vi "LaneExtractorHenes.vi"() -> ()   [LabVIEW 2024]
uses:
  <vilib>/userDefined/High Color/IMAQdx.ctl
  <vilib>/Instr/_visa.llb/VISA Set IO Buffer Mask.ctl
  <vilib>/Instr/_visa.llb/VISA Flush IO Buffer Mask.ctl
  <vilib>/Python/Open Venv Python Session.vi
  <vilib>/Instr/_visa.llb/VISA Configure Serial Port (Instr).vi
  <vilib>/vision/driver/NI_Vision_Acquisition_Software.lvlib
panel:
  out "inference time":string
  out "error out 3":errorcluster
  out "Image_String":string
  in  "File Path":path=path "C:/Users/JungiHong/OneDrive/Hongik/HI-RACE/2026-01/platform_1_5/ExperimentModules/LaneTracking/forTrainImages/frame_021.jpg"
  in  "UseVideo":bool
  in  "Cam No.":T1="cam3"
  out "Debug":T2(plugin-control)
  in  "input_spd":i16
  in  "HENES":refnum<visa-resource-name>="COM5"
  out "E-STOP":bool
  out "Remote_M/A":bool
  out "Steer_Feed":dbl
  out "Alive_PCU":u8(slide) scale=0.0..254.0
  out "Gear_Feed":u8
  out "Speed_Feed(RPM)":dbl format="%#_g rpm"
  out "버퍼 읽기":string
  out "Speed_Feed(m/s)":dbl
  in  "HLV_Gear":u8
  in  "HLV_A/M":bool=TRUE
  in  "HLV_E-stop":bool
  out "HENES Loop Time":u32=21
  in  "v(Velocity)m/s":dbl=1.0
  in  "k(Gain)":dbl=1.0
  out "δ(OutputSteer)degrees":dbl=6.391264837490994
  in  "max_rmse":u32=1000
  in  "min_span":u32=4
  in  "min_area":u32=4
  out "Right":T2(plugin-control)
  out "changearray":u32=3
  out "CV Loop Time":u32=32
  out "error out 2":errorcluster
  out "error out":errorcluster
  out "return value":string[](array[string])=["0.0", "0.11201359920254694", "C:\\Users\\JungiHong\\OneDrive\\Hongik\\HI-RACE\\2026-01\\platform_1_5\\ExperimentModules\\LaneTracking\\DebugImageFolder\\left_lane.png", "C:\\Users\\JungiHong\\OneDrive\\Hongik\\HI-RACE\\2026-01\\platform_1_5\\ExperimentModules\\LaneTracking\\DebugImageFolder\\right_lane.png", "C:\\Users\\JungiHong\\OneDrive\\Hongik\\HI-RACE\\2026-01\\platform_1_5\\ExperimentModules\\LaneTracking\\DebugImageFolder\\debug_image.png"]
  out "python_error":errorcluster
  out "Left":T2(plugin-control)
  in  "stop":bool
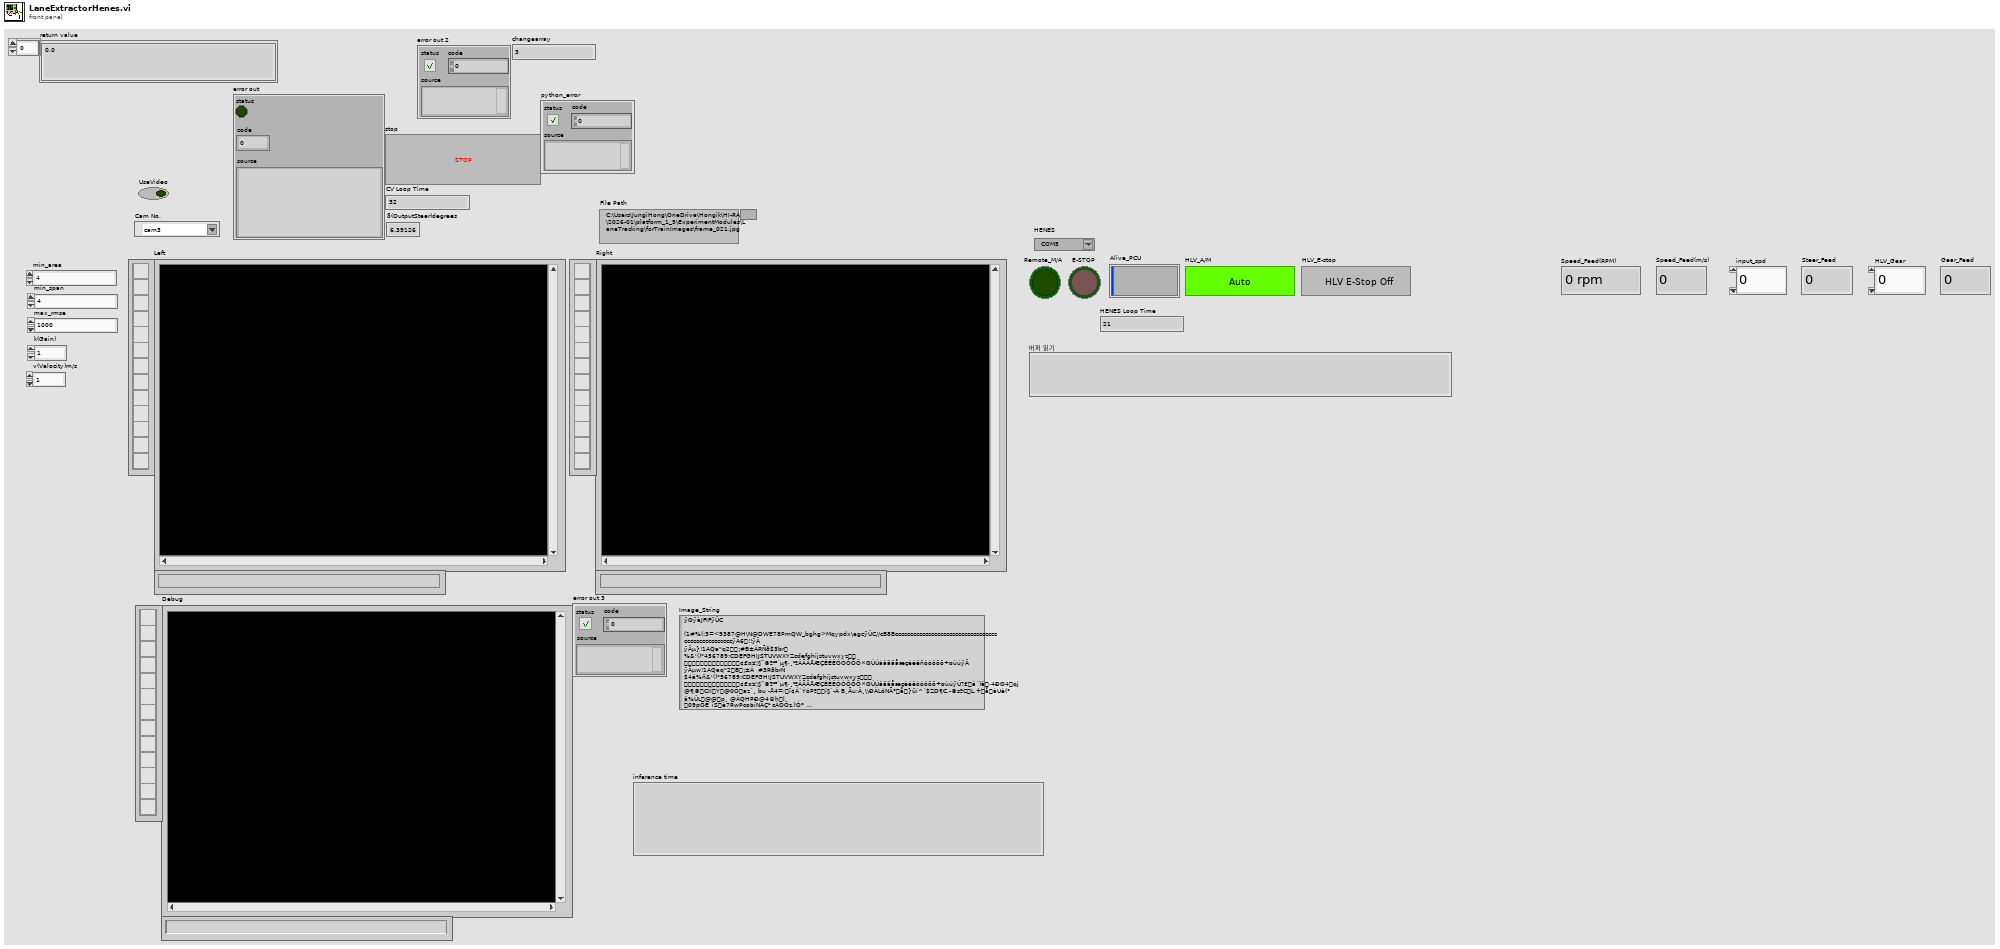
[diagram p1: front panel]
types:
  T1 = typedef "IMAQdx.ctl" = refnum<k21>
  T2 = typedef "IMAQ Image.ctl" = refnum<image>
  T3 = cluster{"HENES_M/A":u8, "HENES_E-Stop":u8, "HENES_Gear":u8, "HENES_Speed":i16, "HENES_Steer":i16, "HENES_Alive":u8}
  T4 = typedef "VISA Flush IO Buffer Mask.ctl" = u16
  T5 = typedef "VISA Set IO Buffer Mask.ctl" = u16
  T6 = cluster{"HLV_M/A_Status":u8, "HLV_E-Stop":u8, "HLV_Gear":u8, "HLV_Speed":i16, "HLV_Steer":i16, "HLV_Alive":u8}
  T7 = cluster{"Global Rectangle":i32[], "Contours":cluster{"ID":enum32{"External", "Internal"}, "Type":u32, "Coordinates":i32[]}[]}
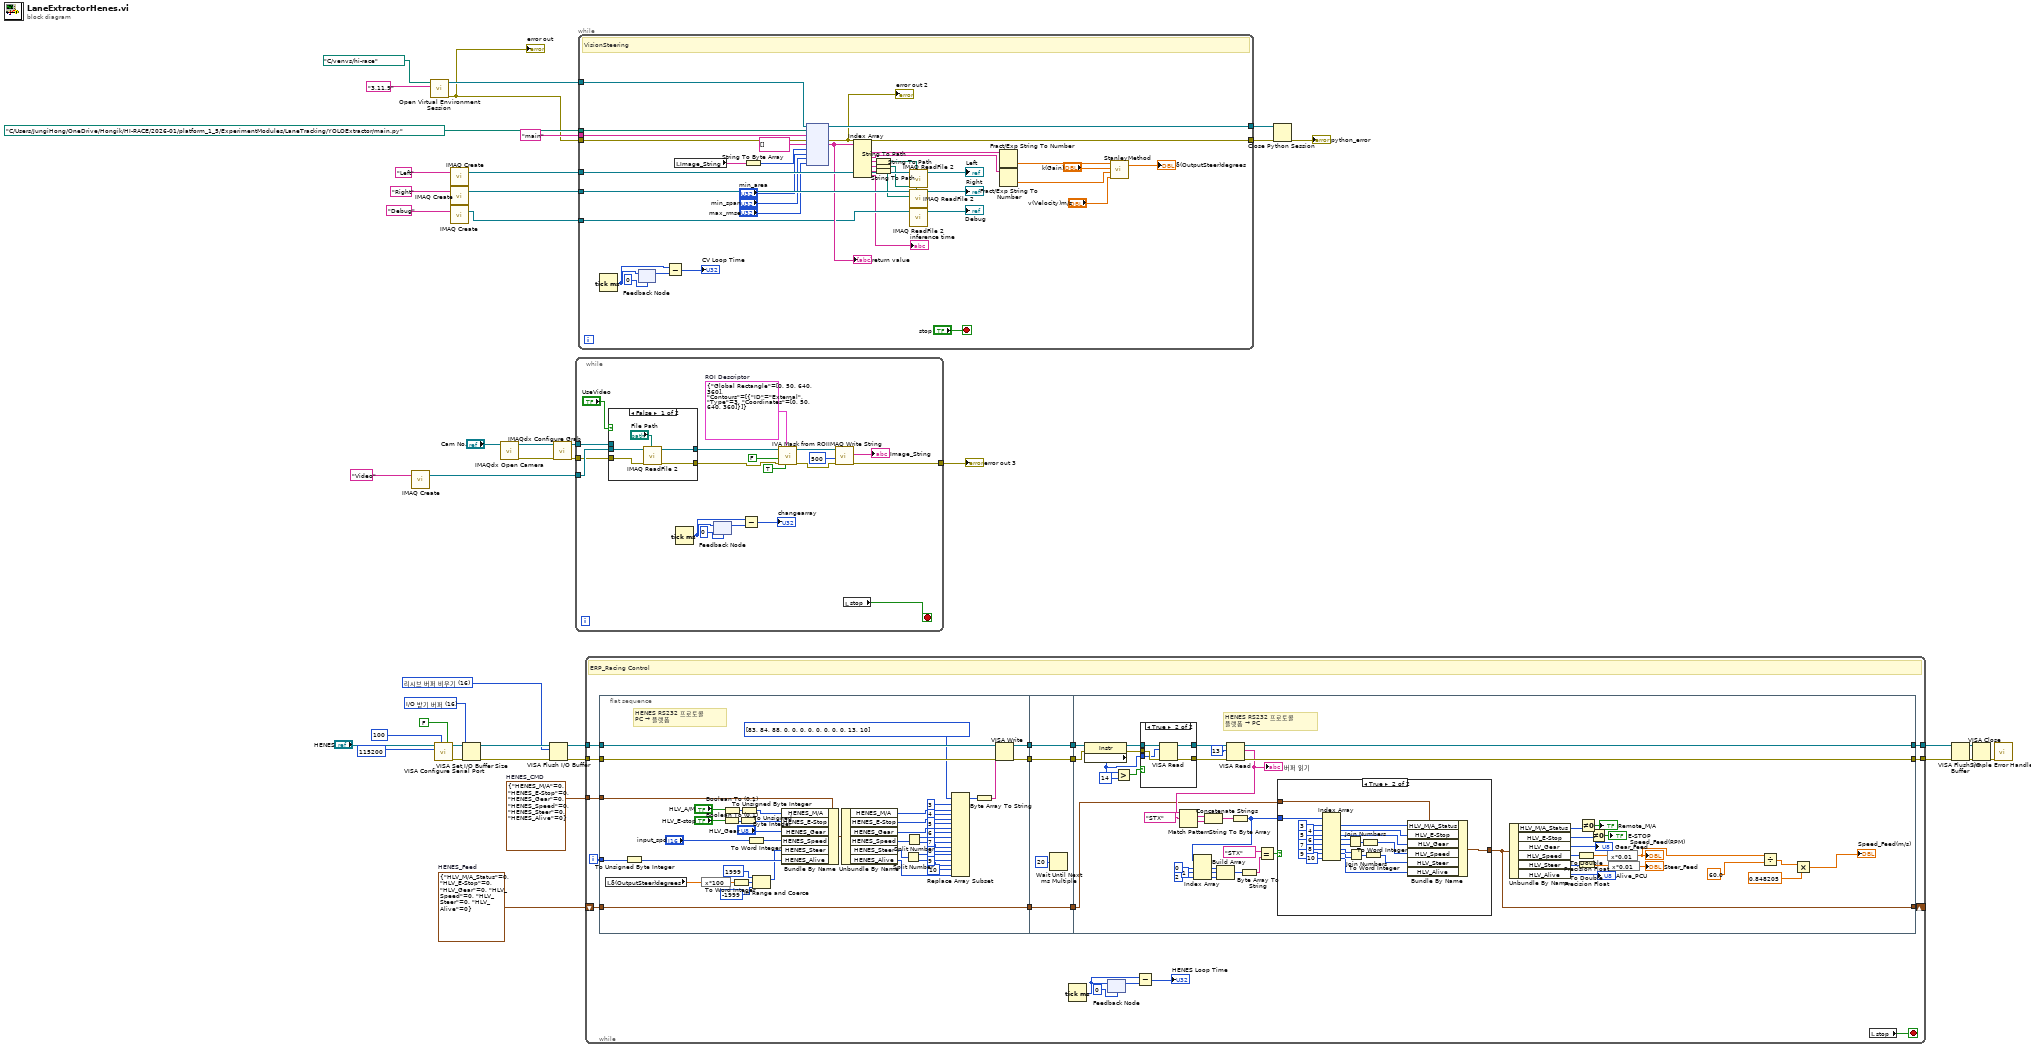
[diagram p0: block diagram]
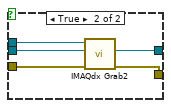
[diagram p4: hidden frame]
diagram:
  w10 = T3 {"HENES_M/A"=0, "HENES_E-Stop"=0, "HENES_Gear"=0, "HENES_Speed"=0, "HENES_Steer"=0, "HENES_Alive"=0}  # HENES_CMD
  w13 = T4 16 items=["리시브 버퍼 비우기"=16, "전달 버퍼 디바이스에 쓰기"=32, "리시브 버퍼 비우기(I/O 없음)"=64, "전달 버퍼 비우기"=128] ("Mask")
  w16 = T5 16 items=["I/O 받기 버퍼"=16, "I/O 전달 버퍼"=32, "I/O 받기와 전달 버퍼"=48] ("Mask")
  w20 = T6 {"HLV_M/A_Status"=0, "HLV_E-Stop"=0, "HLV_Gear"=0, "HLV_Speed"=0, "HLV_Steer"=0, "HLV_Alive"=0}  # HENES_Feed
  n1 = call "IMAQ Create"("Image Name"="Video") -> ("New Image"=w30:T2)  [unwired: 4 in, 1 out]
  n2 = call-poly <vilib>:"Open Virtual Environment Session.vi"("Python version"="3.11.9", "Env path"=path "C:/venvs/hi-race") -> ("error out"=w32:errorcluster, "session out"=w42:refnum<k35>)  [unwired: 8 in]
  "error out" <- w32
  n3 = call-poly "VISA Configure Serial Port"("VISA resource name"="HENES", "timeout (10sec)"=u32 100, "Enable Termination\nChar (T)"=FALSE ("Enable Termination\nChar (T)"), "baud rate (9600)"=u32 115200) -> ("VISA resource name out"=w12:refnum<visa-resource-name>, "error out"=w11:errorcluster)  [unwired: 10 in]
  n4 = call "IMAQ Create"("Image Name"="Left") -> ("New Image"=w37:T2)  [unwired: 4 in, 1 out]
  n5 = call "IMAQ Create"("Image Name"="Right") -> ("New Image"=w28:T2)  [unwired: 4 in, 1 out]
  n6 = call "IMAQ Create"("Image Name"="Debug") -> ("New Image"=w7:T2)  [unwired: 4 in, 1 out]
  n7 = VISA Set I/O Buffer Size(VISA resource name=w12, mask (16)=w16, error in (no error)=w11) -> (VISA resource name out=w15:refnum<visa-resource-name>, error out=w14:errorcluster)  [unwired: 1 in]
  n8 = call <vilib>:"IMAQdx Open Camera.vi"("Session In"="Cam No.") -> ("error out"=w4:errorcluster, "Session Out"=w5:T1)  [unwired: 9 in]
  n9 = VISA Flush I/O Buffer(VISA resource name=w15, mask (16)=w13, error in (no error)=w14) -> (VISA resource name out=w25:refnum<visa-resource-name>, error out=w24:errorcluster)
  n10 = call <vilib>:"IMAQdx Configure Grab.vi"("error in"=w4, "Session In"=w5) -> ("error out"=w3:errorcluster, "Session Out"=w6:T1)  [unwired: 8 in]
  n11 = while {
    tunnel: w30 -> [w56]
    tunnel: w6 -> [w55]
    tunnel: w3 -> [w54]
    tunnel: [w46] -> w1
    stop <- w61 stop-if-true
    w51 = T7 {"Global Rectangle"=[0, 50, 640, 360], "Contours"=[{"ID"=enum."External", "Type"=3, "Coordinates"=[0, 50, 640, 360]}]}  # ROI Descriptor
    n12 = case shown="False" "UseVideo" {
      tunnel: w56 -> [w64 w71]
      tunnel: [w66 w70] -> w44
      tunnel: [w65 w69] -> w49
      tunnel: w55 -> [_ w68]
      tunnel: w54 -> [w62 w67]
      frame False {
        n13 = call "IMAQ ReadFile 2"("File Path"="File Path", "error in (no error)"=w62, "Image"=w64) -> ("error out"=w66:errorcluster, "Image Out"=w65:T2)  [unwired: 4 in, 3 out]
      }
      frame True {
        n14 = call <vilib>:"IMAQdx Grab2.vi"("error in"=w67, "Image In"=w71, "Session In"=w68) -> ("error out"=w70:errorcluster, "Image Out"=w69:T2)  [unwired: 5 in, 2 out]
      }
    }
    n15 = Tick Count (ms)() -> (millisecond timer value=w57:u32)
    n16 = feedback #1(u32 0 ("millisecond timer value")) -> (w58:u32)
    n17 = feedback-in #1(w57) -> ()
    n18 = Subtract(x=w57, y=w58) -> (x-y=→"changearray":u32)
    n19 = call <vilib>:"IVA Mask from ROI.vi"("Shrink"=TRUE, "ROI Descriptor"=w51, "error in (no error)"=w44, "Out / In"=FALSE, "Image Src"=w49) -> ("error out"=w43:errorcluster, "Image Out"=w47:T2)  [unwired: 5 out]
    n20 = call-poly "IMAQ Write String"("error in (no error)"=w43, "Image Quality"=u32 500, "Image"=w47) -> ("error out"=w46:errorcluster, "FileString"=→"Image_String":string)  [unwired: 6 in, 1 out]
    n21 = local read "stop"() -> (w61:bool)
  }
  "error out 3" <- w1
  n22 = while {
    tunnel: w42 -> [w108]
    tunnel: [w107] -> w39
    tunnel: w37 -> [w101]
    tunnel: path "C:/Users/JungiHong/OneDrive/Hongik/HI-RACE/2026-01/platform_1_5/ExperimentModules/LaneTracking/YOLOExtractor/main.py" ("module in") -> [w105]
    tunnel: "main" ("module out") -> [w104]
    tunnel: w32 -> [w103]
    tunnel: [w102] -> w34
    tunnel: w28 -> [w93]
    tunnel: w7 -> [w78]
    stop <- "stop" stop-if-true
    # "VisionSteering"
    n23 = Tick Count (ms)() -> (millisecond timer value=w98:u32)
    n24 = feedback #2(u32 0 ("millisecond timer value")) -> (w97:u32)
    n25 = feedback-in #2(w98) -> ()
    n26 = Subtract(x=w98, y=w97) -> (x-y=→"CV Loop Time":u32)
    n27 = local read "Image_String"() -> (w74:string)
    n28 = String To Byte Array(string=w74) -> (unsigned byte array=w73:u8[])
    n29 = node(w108, w105, w104, w103, string[] [], w73, "min_area", "min_span", "max_rmse") -> (w107:refnum<k35>, w102:errorcluster, w92:string[])  [unwired: 4 in, 2 out]
    "return value" <- w92
    "error out 2" <- w102
    n30 = Index Array(array=w92) -> (element #1=w88:string, element #2=w87:string, element #3=w90:string, element #4=w89:string, element #5=w80:string, element #6=→"inference time":string)  [unwired: 6 in]
    n31 = String To Path(string=w90) -> (path=w99:path)
    n32 = String To Path(string=w89) -> (path=w91:path)
    n33 = String To Path(string=w80) -> (path=w79:path)
    n34 = call "IMAQ ReadFile 2"("File Path"=w99, "Image"=w101) -> ("Image Out"=→"Left":T2)  [unwired: 5 in, 4 out]
    n35 = call "IMAQ ReadFile 2"("File Path"=w91, "Image"=w93) -> ("Image Out"=→"Right":T2)  [unwired: 5 in, 4 out]
    n36 = call "IMAQ ReadFile 2"("File Path"=w79, "Image"=w78) -> ("Image Out"=→"Debug":T2)  [unwired: 5 in, 4 out]
    n37 = Fract/Exp String To Number(string=w88) -> (number=w85:dbl)  [unwired: 3 in, 1 out]
    n38 = Fract/Exp String To Number(string=w87) -> (number=w84:dbl)  [unwired: 3 in, 1 out]
    n39 = call "StanleyMethod.vi"("v(Velocity)m/s"="v(Velocity)m/s", "e(Cross-Track Err)m/s"=w84, "k(Gain)"="k(Gain)", "ψ(Heading Err)radian"=w85) -> ("δ(OutputSteer)degrees"=→"δ(OutputSteer)degrees":dbl)  [unwired: 1 out]
  }
  n40 = while {
    tunnel: w25 -> [w128]
    tunnel: w24 -> [w127]
    tunnel: [w121] -> w23
    tunnel: [w120] -> w22
    shift-right: [w115] -> _
    shift-left: w20 -> [w118]
    tunnel: w10 -> [w116]
    i -> [w122]
    stop <- w110 stop-if-true
    # "ERP_Racing Control"
    n41 = flat-sequence {
      tunnel: [w171] -> w125
      tunnel: [w170] -> w123
      tunnel: w128 -> [w173]
      tunnel: w127 -> [w172]
      tunnel: w122 -> [w169]
      tunnel: [w168] -> w119
      tunnel: w118 -> [w168]
      tunnel: w116 -> [w167]
      tunnel: [w177] -> w126
      tunnel: w125 -> [w177]
      tunnel: [w176] -> w124
      tunnel: w123 -> [w176]
      tunnel: w119 -> [w174]
      tunnel: [w174] -> w117
      tunnel: w126 -> [w205]
      tunnel: w124 -> [w204]
      tunnel: [w222] -> w121
      tunnel: [w221] -> w120
      tunnel: w117 -> [w196]
      tunnel: [w194] -> w115
      frame #0 {
        # "HENES RS232 프로토콜\nPC → 플랫폼"
        n42 = local read "δ(OutputSteer)degrees"() -> (w129:dbl)
        n43 = To Unsigned Byte Integer(number=w169) -> (unsigned 8bit integer=w156:u8)
        n44 = expression code="x*100"(w129) -> (w131:dbl)
        n45 = Boolean To (0,1)(Boolean="HLV_E-stop") -> (0, 1=w151:i16)
        n46 = Boolean To (0,1)(Boolean="HLV_A/M") -> (0, 1=w152:i16)
        n47 = To Word Integer(number=w131) -> (16bit integer=w134:i16)
        n48 = To Unsigned Byte Integer(number=w151) -> (unsigned 8bit integer=w149:u8)
        n49 = To Unsigned Byte Integer(number=w152) -> (unsigned 8bit integer=w150:u8)
        n50 = To Word Integer(number="input_spd") -> (16bit integer=w143:i16)
        n51 = In Range and Coerce(upper limit=i16 1999 ("상위 리미트"), x=w134, lower limit=i16 -1999 ("상위 리미트")) -> (coerced(x)=w142:i16)  [unwired: 1 out]
        n52 = Bundle By Name(cluster=w167, "HENES_M/A"=w150, "HENES_E-Stop"=w149, "HENES_Gear"="HLV_Gear", "HENES_Speed"=w143, "HENES_Steer"=w142, "HENES_Alive"=w156) -> (w160:T3)
        n53 = Unbundle By Name(w160) -> ("HENES_M/A"=w146:u8, "HENES_E-Stop"=w145:u8, "HENES_Gear"=w135:u8, "HENES_Speed"=w138:i16, "HENES_Steer"=w141:i16, "HENES_Alive"=w155:u8)
        n54 = Split Number(x=w141) -> (hi(x)=w140:u8, lo(x)=w139:u8)
        n55 = Split Number(x=w138) -> (hi(x)=w137:u8, lo(x)=w136:u8)
        n56 = Replace Array Subset(array=u8[] [83, 84, 88, 0, 0, 0, 0, 0, 0, 0, 0, 13, 10] ("unsigned byte array"), new element #1=w146, index #1=3, new element #2=w145, index #2=4, new element #3=w135, index #3=5, new element #4=w137, index #4=6, new element #5=w136, index #5=7, new element #6=w140, index #6=8, new element #7=w139, index #7=9, new element #8=w155, index #8=10) -> (w158:u8[])
        n57 = Byte Array To String(unsigned byte array=w158) -> (string=w157:string)
        n58 = VISA Write(VISA resource name=w173, write buffer=w157, error in (no error)=w172) -> (VISA resource name out=w171:refnum<visa-resource-name>, error out=w170:errorcluster)  [unwired: 1 out]
      }
      frame #1 {
        n59 = Wait Until Next ms Multiple(millisecond multiple=u32 20 ("대기 시간 (ms)")) -> ()  [unwired: 1 out]
      }
      frame #2 {
        # "HENES RS232 프로토콜\n플랫폼 → PC"
        n60 = property class="Instr"(reference=w205, error in=w204) -> (reference out=w185:refnum<visa-resource-name>, error out=w184:errorcluster, "Serial Settings:Number of Bytes at Serial Port"=w183:u32)
        n61 = Greater?(x=w183, y=u32 14) -> (0:w201:bool)
        n62 = case shown="True" w201 {
          tunnel: w185 -> [w249 w254]
          tunnel: w184 -> [w248 w253]
          tunnel: [w249 w252] -> w203
          tunnel: [w248 w251] -> w202
          tunnel: w183 -> [_ w250]
          frame False {
          }
          frame True {
            n63 = VISA Read(VISA resource name=w254, byte count=w250, error in (no error)=w253) -> (VISA resource name out=w252:refnum<visa-resource-name>, error out=w251:errorcluster)  [unwired: 2 out]
          }
        }
        n64 = VISA Read(VISA resource name=w203, byte count=u32 13, error in (no error)=w202) -> (VISA resource name out=w222:refnum<visa-resource-name>, read buffer=w220:string, error out=w221:errorcluster)  [unwired: 1 out]
        "버퍼 읽기" <- w220
        n65 = Match Pattern(string=w220, regular expression="STX") -> (match substring=w217:string, after substring=w218:string)  [unwired: 1 in, 2 out]
        n66 = Concatenate Strings(w217, w218) -> (w216:string)
        n67 = String To Byte Array(string=w216) -> (unsigned byte array=w198:u8[])
        n68 = Index Array(array=w198, index #1=0, index #2=1, index #3=2) -> (element #1=w211:u8, element #2=w210:u8, element #3=w209:u8)
        n69 = Build Array(w211, w210, w209) -> (w208:u8[])
        n70 = Byte Array To String(unsigned byte array=w208) -> (string=w206:string)
        n71 = Equal?(x="STX", y=w206) -> (x = y?=w197:bool)
        n72 = case shown="True" w197 {
          tunnel: w198 -> [_ w247]
          tunnel: [w224 w234] -> w194
          tunnel: w196 -> [w224 w236]
          frame False {
          }
          frame True {
            n73 = Index Array(array=w247, index #1=3, index #2=4, index #3=5, index #4=6, index #5=7, index #6=8, index #7=9, index #8=10) -> (element #1=w235:u8, element #2=w233:u8, element #3=w232:u8, element #4=w231:u8, element #5=w230:u8, element #6=w228:u8, element #7=w227:u8, element #8=w225:u8)
            n74 = Join Numbers(hi=w231, lo=w230) -> ((hi.lo)=w238:u16)
            n75 = Join Numbers(hi=w228, lo=w227) -> ((hi.lo)=w237:u16)
            n76 = To Word Integer(number=w238) -> (16bit integer=w229:i16)
            n77 = To Word Integer(number=w237) -> (16bit integer=w226:i16)
            n78 = Bundle By Name(cluster=w236, "HLV_M/A_Status"=w235, "HLV_E-Stop"=w233, "HLV_Gear"=w232, "HLV_Speed"=w229, "HLV_Steer"=w226, "HLV_Alive"=w225) -> (w234:T6)
          }
        }
        n79 = Unbundle By Name(w194) -> ("HLV_M/A_Status"=w195:u8, "HLV_E-Stop"=w189:u8, "HLV_Gear"=→"Gear_Feed":u8, "HLV_Speed"=w187:i16, "HLV_Steer"=w186:i16, "HLV_Alive"=→"Alive_PCU":u8)
        n80 = To Double Precision Float(number=w187) -> (double precision float=w199:dbl)
        n81 = To Double Precision Float(number=w186) -> (double precision float=w192:dbl)
        n82 = Not Equal To 0?(x=w195) -> (x != 0?=→"Remote_M/A":bool)
        n83 = Not Equal To 0?(x=w189) -> (x != 0?=→"E-STOP":bool)
        n84 = expression code="x*0.01"(w199) -> (w178:dbl)
        "Speed_Feed(RPM)" <- w178
        n85 = expression code="x*0.01"(w192) -> (→"Steer_Feed":dbl)
        n86 = Divide(x=w178, y=60.0) -> (x/y=w182:dbl)
        n87 = Multiply(x=w182, y=0.848205) -> (x*y=→"Speed_Feed(m/s)":dbl)
      }
    }
    n88 = Tick Count (ms)() -> (millisecond timer value=w112:u32)
    n89 = feedback #3(u32 0 ("millisecond timer value")) -> (w113:u32)
    n90 = feedback-in #3(w112) -> ()
    n91 = Subtract(x=w112, y=w113) -> (x-y=→"HENES Loop Time":u32)
    n92 = local read "stop"() -> (w110:bool)
  }
  n93 = Close Python Session(session in=w39, error in=w34) -> (11:→"python_error":errorcluster)
  n94 = VISA Flush I/O Buffer(VISA resource name=w23, error in (no error)=w22) -> (VISA resource name out=w26:refnum<visa-resource-name>, error out=w27:errorcluster)  [unwired: 1 in]
  n95 = VISA Close(VISA resource name=w26, error in (no error)=w27) -> (error out=w21:errorcluster)
  n96 = call <vilib>:"Simple Error Handler.vi"("error in (no error)"=w21) -> ()  [unwired: 4 in, 5 out]
